vi "控件配置文件.vi"() -> ()   [LabVIEW 2018]
panel:
  out "控件配置文件":string[][](table)
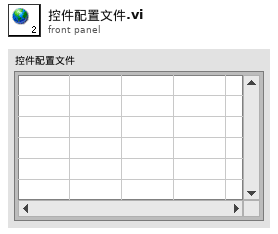
[diagram p1: front panel]
diagram:
